vi "Set Finger Angles.vi"(8 "error in (no error)":errorcluster, 11 "MF3 in":refnum<class "MF3.lvclass">) -> (0 "error out":errorcluster, 3 "MF3 out":refnum<class "MF3.lvclass">)   [LabVIEW 2013, in "MF3.lvclass"]
uses:
  MF3.lvclass
  controls/Motor Names.ctl
  MF3.lvclass/MF3.ctl
  Finger/Finger.lvclass
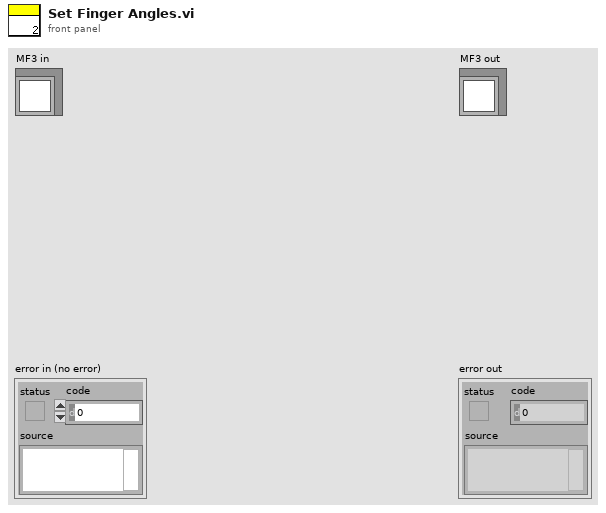
[diagram p1: front panel]
types:
  T1 = typedef "Motor Names.ctl" = enum16{"Thumb1", "Thumb2", "Thumb3", "Middle1", "Middle2", "Middle3", "Redundant", "Index1", "Index2", "Index3"}
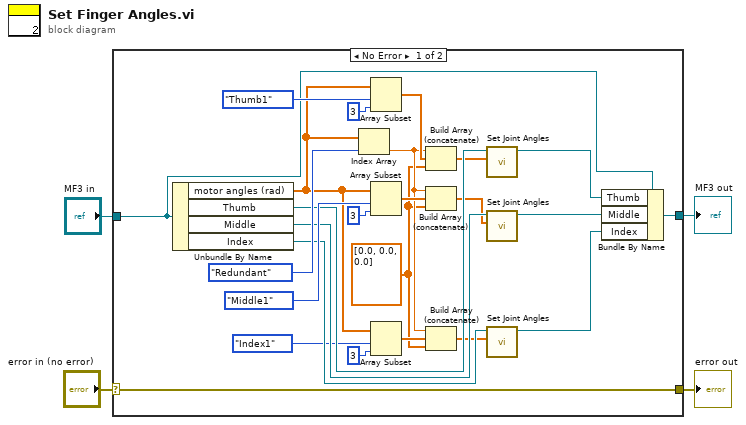
[diagram p0: block diagram]
diagram:
  n1 = case shown="No Error" "error in (no error)" {
    selector: "error in (no error)" -> [w29 w31]
    tunnel: [w29 w31] -> w3
    tunnel: [w10 w30] -> w1
    tunnel: "MF3 in" -> [w14 w30]
    frame No Error {
      w5 = dbl[] [0.0, 0.0, 0.0] ("subarray")
      n2 = Unbundle By Name(w14) -> ("motor angles (rad)"=w18:dbl[], "Thumb"=w17:refnum<class "Finger.lvclass">, "Middle"=w16:refnum<class "Finger.lvclass">, "Index"=w15:refnum<class "Finger.lvclass">)
      n3 = Index Array(array=w18, index=Motor_Names."Redundant" ("Motor Names")) -> (element=w19:dbl)
      n4 = Array Subset(array=w18, index=Motor_Names."Thumb1" ("Motor Names"), length=3) -> (w26:dbl[])
      n5 = Array Subset(array=w18, index=Motor_Names."Middle1" ("Motor Names"), length=3) -> (w24:dbl[])
      n6 = Array Subset(array=w18, index=Motor_Names."Index1" ("Motor Names"), length=3) -> (w21:dbl[])
      n7 = Build Array (concatenate)(w19, w26, w5) -> (w6:dbl[])
      n8 = Build Array (concatenate)(w19, w24, w5) -> (w7:dbl[])
      n9 = Build Array (concatenate)(w19, w21, w5) -> (w8:dbl[])
      n10 = call "Set Joint Angles.vi"("motor_angles"=w6, "Finger in"=w17) -> ("Finger out"=w13:refnum<class "Finger.lvclass">)  [unwired: 8 in, 1 out]
      n11 = call "Set Joint Angles.vi"("motor_angles"=w7, "Finger in"=w16) -> ("Finger out"=w12:refnum<class "Finger.lvclass">)  [unwired: 8 in, 1 out]
      n12 = call "Set Joint Angles.vi"("motor_angles"=w8, "Finger in"=w15) -> ("Finger out"=w11:refnum<class "Finger.lvclass">)  [unwired: 8 in, 1 out]
      n13 = Bundle By Name(cluster=w14, "Thumb"=w13, "Middle"=w12, "Index"=w11) -> (w10:refnum<class "MF3.lvclass">)
    }
    frame Error {
    }
  }
  "error out" <- w3
  "MF3 out" <- w1
